vi "Leap Motion - Keytap shape data.vi"(8 "Error In":errorcluster, 10 "Key tap":string[](array[string])) -> (0 "Error Out":errorcluster, 2 "Keytap cluster":T1)   [LabVIEW 2014]
uses:
  Typedef/keytap_data.ctl
panel:
  in  "Keytap data":T1
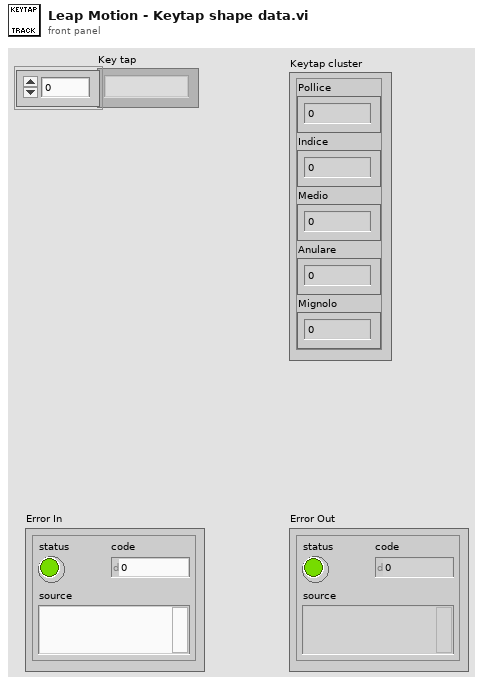
[diagram p1: front panel]
types:
  T1 = typedef "keytap_data.ctl" = cluster{"Pollice":u8, "Indice":u8, "Medio":u8, "Anulare":u8, "Mignolo":u8}
  T2 = cluster{"Key tap[0]":string, "Key tap[1]":string, "Key tap[2]":string, "Key tap[3]":string, "Key tap[4]":string}
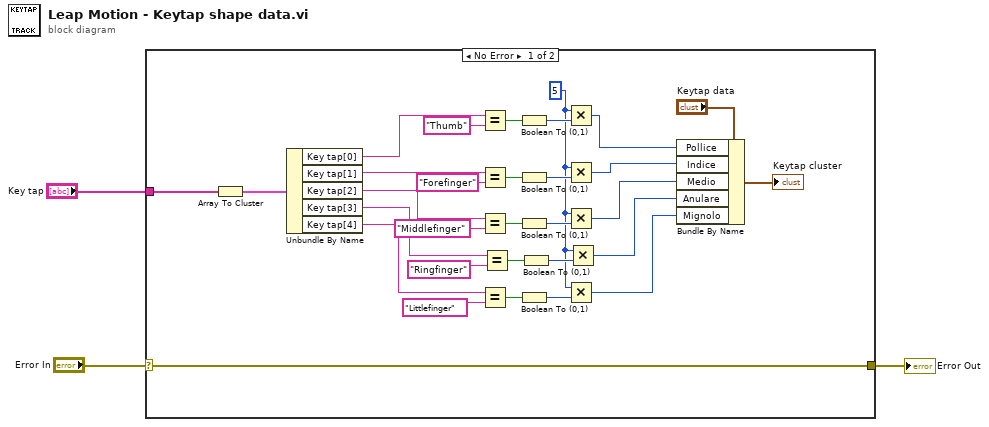
[diagram p0: block diagram]
diagram:
  n1 = case shown="No Error" "Error In" {
    selector: "Error In" -> [w11 w35]
    tunnel: "Key tap" -> [w34 _]
    tunnel: [w11 w35] -> w1
    frame No Error {
      w12 = i16 5 ("x")
      n2 = Array To Cluster(array=w34) -> (cluster=w33:T2)
      n3 = Unbundle By Name(w33) -> ("Key tap[0]"=w32:string, "Key tap[1]"=w20:string, "Key tap[2]"=w19:string, "Key tap[3]"=w18:string, "Key tap[4]"=w17:string)
      n4 = Equal?(x=w32, y="Thumb") -> (x = y?=w30:bool)
      n5 = Equal?(x=w20, y="Forefinger") -> (x = y?=w28:bool)
      n6 = Equal?(x=w19, y="Middlefinger") -> (x = y?=w26:bool)
      n7 = Equal?(x=w17, y="Littlefinger") -> (x = y?=w22:bool)
      n8 = Equal?(x=w18, y="Ringfinger") -> (x = y?=w24:bool)
      n9 = Boolean To (0,1)(Boolean=w30) -> (0, 1=w29:i16)
      n10 = Boolean To (0,1)(Boolean=w28) -> (0, 1=w27:i16)
      n11 = Boolean To (0,1)(Boolean=w26) -> (0, 1=w25:i16)
      n12 = Boolean To (0,1)(Boolean=w22) -> (0, 1=w21:i16)
      n13 = Boolean To (0,1)(Boolean=w24) -> (0, 1=w23:i16)
      n14 = Multiply(x=w12, y=w29) -> (x*y=w10:i16)
      n15 = Multiply(x=w12, y=w27) -> (x*y=w9:i16)
      n16 = Multiply(x=w12, y=w25) -> (x*y=w8:i16)
      n17 = Multiply(x=w12, y=w21) -> (x*y=w5:i16)
      n18 = Multiply(x=w12, y=w23) -> (x*y=w7:i16)
      n19 = Bundle By Name(cluster="Keytap data", "Pollice"=w10, "Indice"=w9, "Medio"=w8, "Anulare"=w7, "Mignolo"=w5) -> (→"Keytap cluster":T1)
    }
    frame Error {
    }
  }
  "Error Out" <- w1
